vi "MPM_Sample.vi"() -> ()   [LabVIEW 2017]
uses:
  <vilib>/Utility/file.llb/Write To Spreadsheet File (DBL).vi
  <vilib>/Utility/file.llb/Write Delimited Spreadsheet (string).vi
  LV_IL_Sample/DLL/InstrumentDLL.dll
panel:
  out "MPM":refnum<k24>
  in  "选项卡控件":T1(tab)
  out "lblver4":string
  out "lblseri4":string
  out "lbltype4":string
  out "lblver3":string
  out "lblseri3":string
  out "lbltype3":string
  out "lblver2":string
  out "lblseri2":string
  out "lbltype2":string
  out "lblver1":string
  out "lblseri1":string
  out "lbltype1":string
  out "lblver0":string
  out "lblseri0":string
  out "lbltype0":string
  out "module count":string
  out "Product":string
  out "Serial":string
  out "F/ W Vesion":string
  in  "btnDisconnect":bool
  in  "btnConnect":bool
  in  "Portnumber":i32
  in  "Address/ComPort":string
  in  "Communication":T2(radio)
  in  "GetComport":bool
  in  "ComPort":u16(ring)
  in  "btnSplit":bool
  out "Address":dbl
  out "Board number":dbl
  in  "btnVisa":bool
  in  "Visa String":u16(ring)
  out "txtlan_port":string
  in  "btnGetPort":bool
  out "txtipaddress":string
  in  "btnGetIP":bool
  out "txtsyst_error":string
  in  "btnGetError":bool
  in  "btnGetWavelength":bool
  in  "txtwave_ch":i32 caption="Ch"
  in  "txtwave_slot":i32 caption="Slot"
  in  "btnZeroing":bool
  out "txtreadp_all":string caption="Read Power for each slot"
  in  "txtread_slotall":i32 caption="Slot"
  in  "btnSlot_Power":bool
  out "txt_readp_ch":dbl caption="Read Power for each ch"
  in  "txtread_ch":i32=1 caption="Ch"
  in  "txtread_slot":i32 caption="Slot"
  in  "btnSlot_Ch_Power":bool
  out "txtget_erange":dbl caption="Range for each ch"
  in  "txtget_rangech":i32=1 caption="Ch"
  in  "txtget_rangeslot":i32 caption="Slot"
  out "txtgetrmode":string caption="Range mode for \"READ\""
  in  "btnSlot_Ch_Range":bool
  in  "btnGet":bool
  out "txtget_unit":string caption="Unit"
  out "txtget_avg":dbl caption="Averaging time(msec)"
  out "txtget_wave":dbl caption="Wavelength(nm)"
  out "txtgetrang":i32 caption="Range All"
  in  "Ch":i32
  in  "Slot":i32
  in  "Range for each ch":i32
  in  "btnSetSlot":bool
  in  "Averaging time(msec)":dbl
  in  "btnSetAveraging":bool
  in  "btnSetUnit":bool
  in  "Unit":u16(ring) items=["dBm", "mW"]
  in  "btnSetRangeAll":bool
  in  "Range All":i32
  in  "btnSetRangeMode":bool
  in  "Range mode for \"READ\"":enum16{"Auto", "Manual"}(ring)
  in  "Wavelength(nm)":dbl
  in  "btnSetWavelength":bool
  in  "btnGetSlot":bool
  in  "txte_slot":i32 caption="Slot"
  in  "btnGetch":bool
  in  "txtlog_ch":i32 caption="Ch"
  in  "txtlog_slot":i32 caption="Slot"
  out "txtlog_status":string
  in  "btnStop":bool
  in  "btnStatus":bool
  in  "btnStart":bool
  in  "btnSetFreerun":bool
  in  "cmbfr_tin_mode":enum16{"Internal", "Extarnal"}(ring) caption="Trigger input mode"
  in  "txtfr_range":i32 caption="Range"
  in  "txtfr_point":i32 caption="number of point"
  in  "txtfr_ave":dbl caption="Averaging Time(msec)"
  in  "txtfr_wave":dbl caption="Wavelength(nm)"
  in  "btnSetSweep":bool
  in  "txtsm_range":i32 caption="Range"
  in  "cmbsm_rangemode":enum16{"Auto", "Manual"}(ring) caption="Range mode"
  in  "txtspeed":i32 caption="Speed(nm/sec)"
  in  "txtwavestep":dbl caption="Step wavelenght(nm)"
  in  "txtstopwave":dbl caption="Stop wavelenght(nm)"
  in  "txtstartwave":dbl caption="Start wavelength(nm)"
  in  "txtcon_range":i32 caption="Range"
  in  "cmbcon_rangemode":enum16{"Auto", "Manual"}(ring) caption="Range mode"
  in  "txtcon_point":i32 caption="number of point"
  in  "txtcon_ave":dbl caption="Averaging Time(msec)"
  in  "txtcon_wave":dbl caption="Wavelength(nm)"
  in  "btnSetConst":bool
  in  "btnGetParameter":bool
  out "txtg_speed":dbl caption="Sweep speed(nm)"
  out "txtg_stepwave":dbl caption="Step wavelength(nm)"
  out "txtg_stopwave":dbl caption="Stop wavelength(nm)"
  out "txtg_statwave":dbl caption="Start wavelength(nm)"
  out "txtg_wavelength":dbl caption="Wavelength(nm)"
  out "txtg_settingrange":string caption="Setting Range"
  out "txtg_tinmode":string caption="Trigger input mode"
  out "txtg_rangemode":string caption="Range mode"
  out "txtlog_mode":string caption="SweepMode"
  out "txtg_point":i32 caption="number of point"
  out "txtg_ave":dbl caption="Averaging time"
  # "0. Connect Tool"
  # "1. Connect"
  # "Communication setting"
  # "Information"
  # "Module Information"
  # "Slot0"
  # "Slot1"
  # "Slot2"
  # "Slot3"
  # "Slot4"
  # "Type"
  # "Serial"
  # "Version"
  # "Set"
  # "Get"
  # "Common function"
  # "Const Mode"
  # "Sweep Mode"
  # "FreerunMode"
  # "Common"
  # "Get Parameter"
  # "Sweep mode parameter"
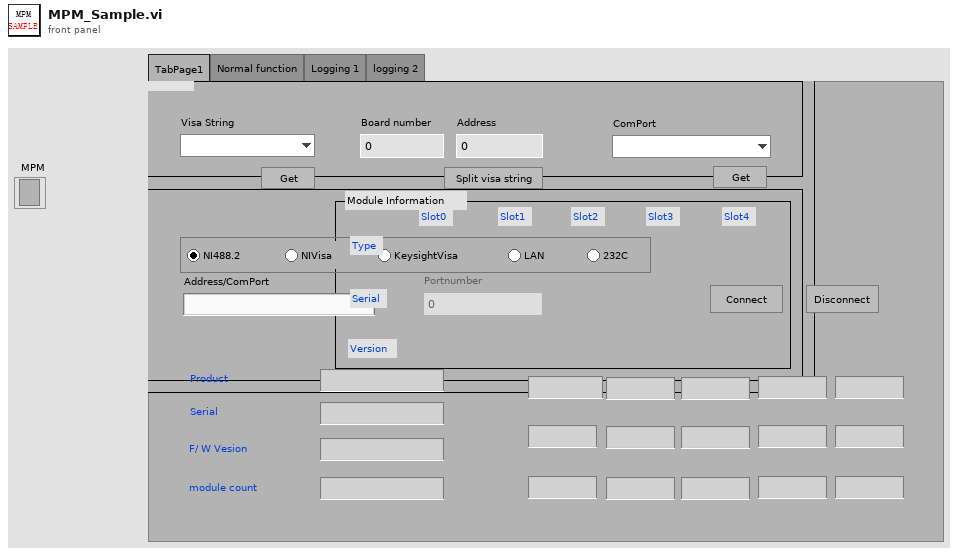
[diagram p1: front panel]
types:
  T1 = enum32{"TabPage1", "Normal function", "Logging 1", "logging 2"}
  T2 = enum32{"rdiNI488", "rdiNIvisa", "rdikeysightvisa", "rdiLAN", "rdi232C"}
  T3 = enum8{"Enabled", "Disabled", "Disabled and Grayed Out"}
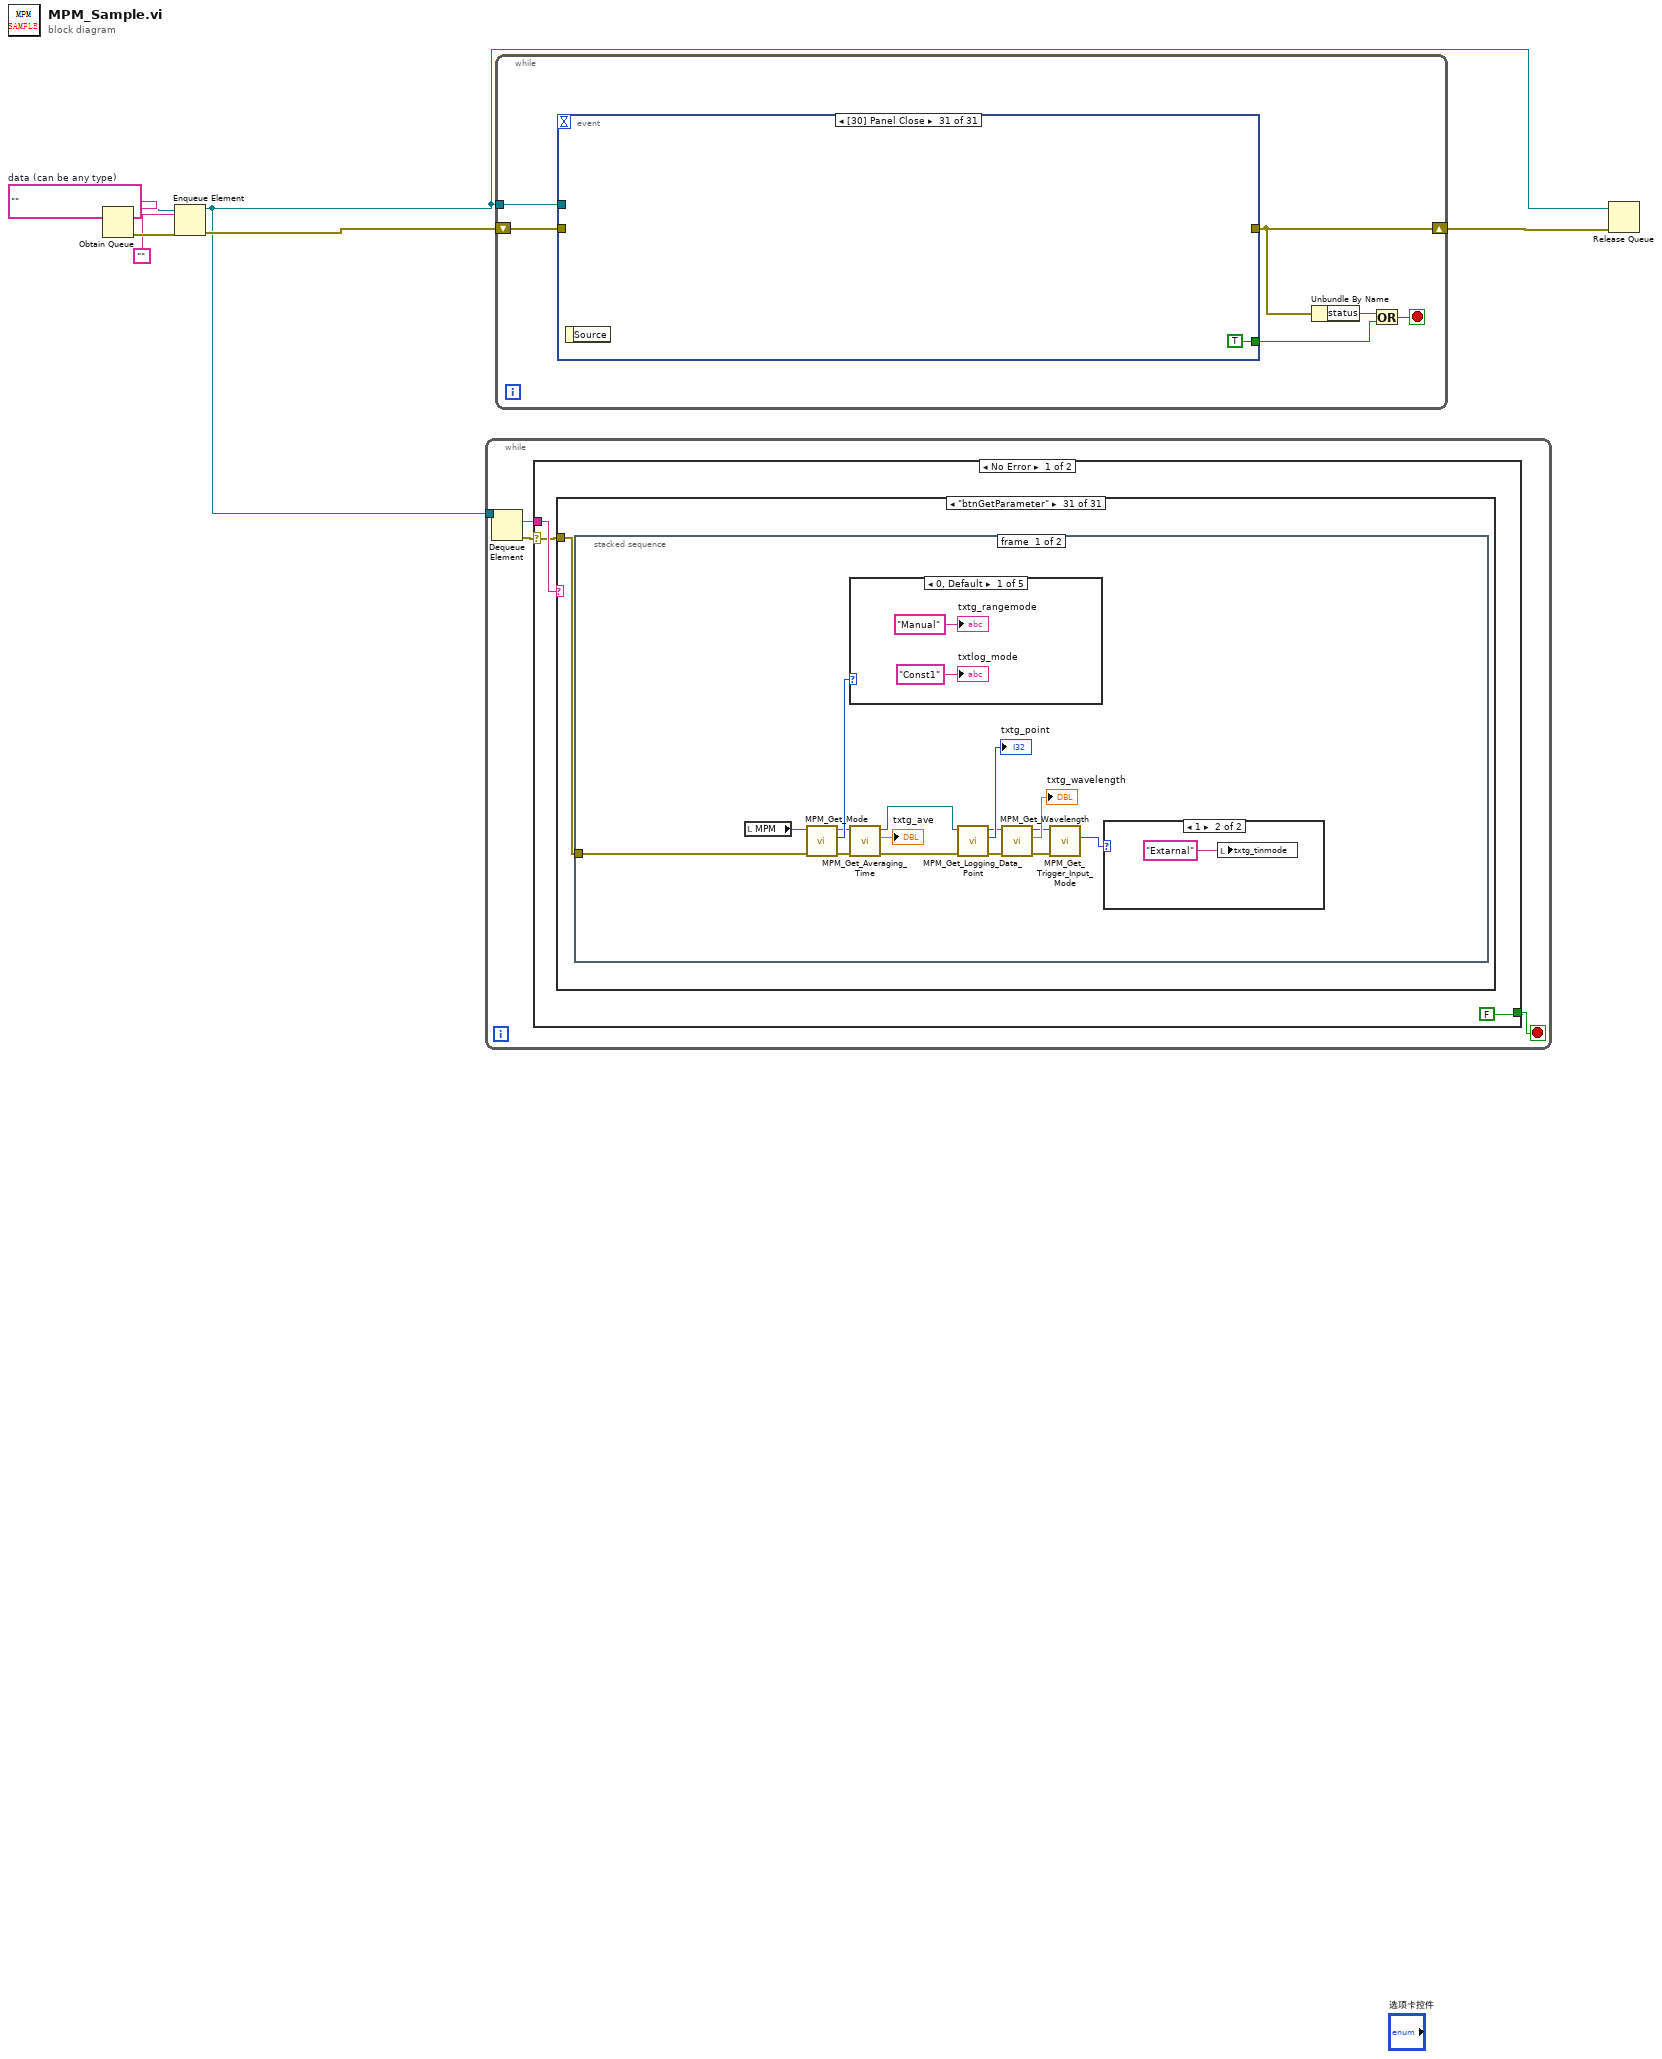
[diagram p0: block diagram]
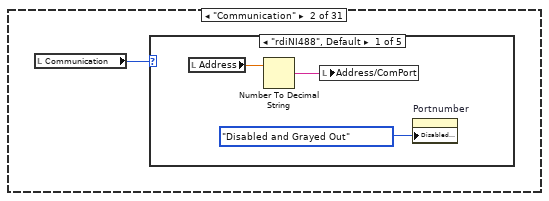
[diagram p3: hidden frame]
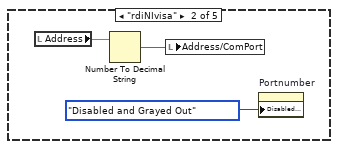
[diagram p4: hidden frame]
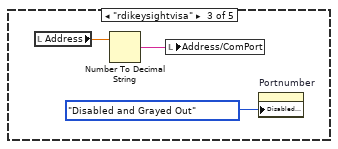
[diagram p5: hidden frame]
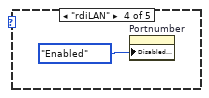
[diagram p6: hidden frame]
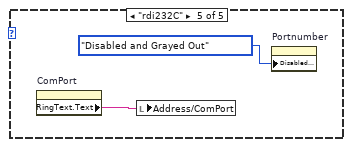
[diagram p7: hidden frame]
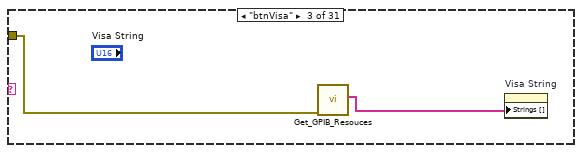
[diagram p8: hidden frame]
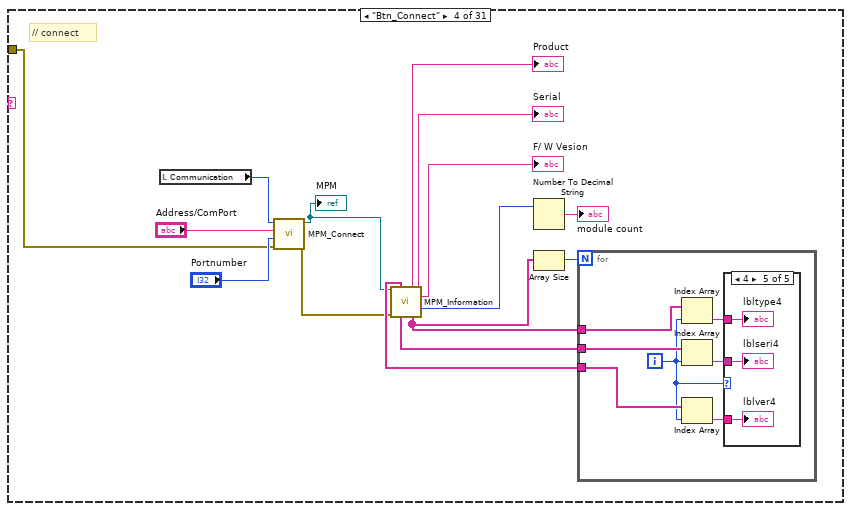
[diagram p9: hidden frame]
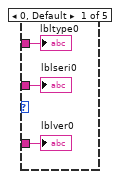
[diagram p10: hidden frame]
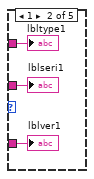
[diagram p11: hidden frame]
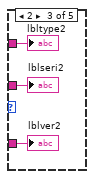
[diagram p12: hidden frame]
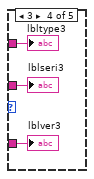
[diagram p13: hidden frame]
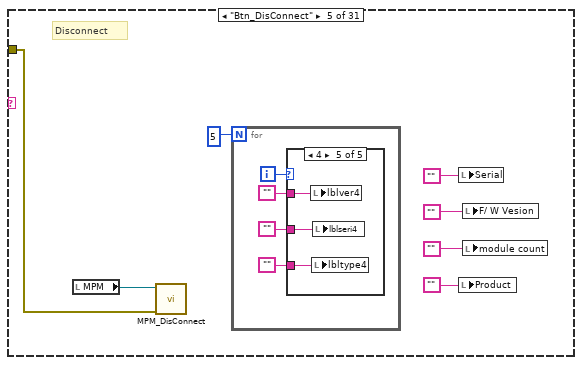
[diagram p14: hidden frame]
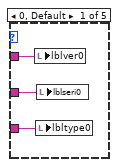
[diagram p15: hidden frame]
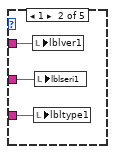
[diagram p16: hidden frame]
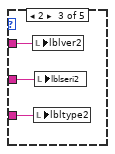
[diagram p17: hidden frame]
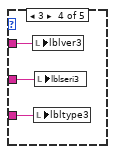
[diagram p18: hidden frame]
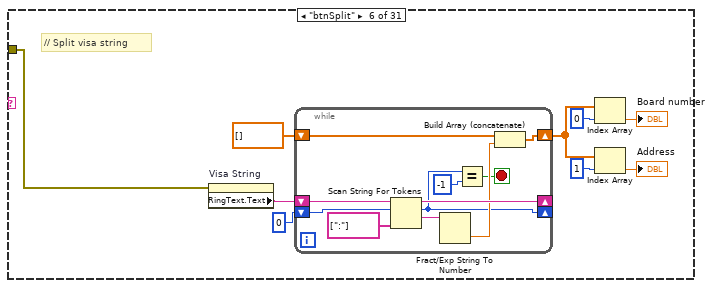
[diagram p19: hidden frame]
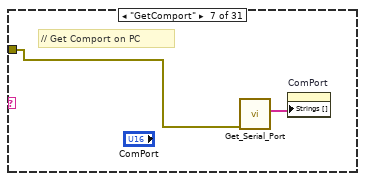
[diagram p20: hidden frame]
diagram:
  w4 = ""  # data (can be any type)
  n1 = Obtain Queue(element data type=w4) -> (queue out=w3:refnum<queue>, error out=w7:errorcluster)  [unwired: 4 in, 1 out]
  n2 = Enqueue Element(queue=w3, element="", error in (no error)=w7) -> (queue out=w1:refnum<queue>, error out=w6:errorcluster)  [unwired: 1 in, 1 out]
  n3 = while {
    tunnel: w1 -> [w11]
    stop <- w8 stop-if-true
    n4 = Dequeue Element(queue=w11) -> (element=w9:string, error out=w10:errorcluster)  [unwired: 2 in, 2 out]
    n5 = case shown="No Error" w10 {
      selector: w10 -> [w12 _]
      tunnel: w9 -> [w13 _]
      tunnel: [FALSE TRUE] -> w8
      frame No Error {
        n6 = case shown="\"btnGetParameter\"" w13 {
          tunnel: w12 -> [_ _ w28 w30 w67 w93 w113 w115 w133 w136 w139 w142 w147 w150 w169 w174 w179 w203 w205 w225 w228 w231 w238 w259 w283 w300 w302 w310 w313 w327 w340]
          frame "Load", Default {
          }
          frame "Communication" {
            n7 = local read "Communication"() -> (w15:T2)
            n8 = case shown="\"rdiNI488\", Default" w15 {
              frame "rdiNI488", Default {
                n9 = local read "Address"() -> (w16:dbl)
                n10 = Number To Decimal String(number=w16) -> (decimal integer string=w17:string)  [unwired: 1 in]
                n11 = local write "Address/ComPort"(w17) -> ()
                n12 = property on="Portnumber" class="DigNum (strict)"("DisabledEnum"=T3."Disabled and Grayed Out" ("禁用")) -> ()  [unwired: 2 in, 2 out]
              }
              frame "rdiNIvisa" {
                n13 = local read "Address"() -> (w19:dbl)
                n14 = Number To Decimal String(number=w19) -> (decimal integer string=w20:string)  [unwired: 1 in]
                n15 = local write "Address/ComPort"(w20) -> ()
                n16 = property on="Portnumber" class="DigNum (strict)"("DisabledEnum"=T3."Disabled and Grayed Out" ("禁用")) -> ()  [unwired: 2 in, 2 out]
              }
              frame "rdikeysightvisa" {
                n17 = local read "Address"() -> (w22:dbl)
                n18 = Number To Decimal String(number=w22) -> (decimal integer string=w23:string)  [unwired: 1 in]
                n19 = local write "Address/ComPort"(w23) -> ()
                n20 = property on="Portnumber" class="DigNum (strict)"("DisabledEnum"=T3."Disabled and Grayed Out" ("禁用")) -> ()  [unwired: 2 in, 2 out]
              }
              frame "rdiLAN" {
                n21 = property on="Portnumber" class="DigNum (strict)"("DisabledEnum"=T3."Enabled" ("禁用")) -> ()  [unwired: 2 in, 2 out]
              }
              frame "rdi232C" {
                n22 = property on="ComPort" class="Ring (strict)"() -> ("RingText.Text"=w26:string)  [unwired: 2 in, 2 out]
                n23 = local write "Address/ComPort"(w26) -> ()
                n24 = property on="Portnumber" class="DigNum (strict)"("DisabledEnum"=T3."Disabled and Grayed Out" ("禁用")) -> ()  [unwired: 2 in, 2 out]
              }
            }
          }
          frame "btnVisa" {
            n25 = call "Get_GPIB_Resouces.vi"("error in (no error)"=w28) -> ("Get_GPIB_Resources"=w29:string[])  [unwired: 8 in, 2 out]
            n26 = property on="Visa String" class="Ring (strict)"("Strings []"=w29) -> ()  [unwired: 2 in, 2 out]
          }
          frame "Btn_Connect" {
            # "// connect"
            n27 = local read "Communication"() -> (w32:T2)
            n28 = call "MPM_Connect.vi"("error in (no error)"=w30, "Portnumber"="Portnumber", "Address/ComPort"="Address/ComPort", "Communication"=w32) -> ("error out"=w33:errorcluster, "Reference out"=w31:refnum<k24>)  [unwired: 6 in]
            "MPM" <- w31
            n29 = call "MPM_Information.vi"(".NET Reference in"=w31, "error in (no error)"=w33) -> ("ModuleFW"=w37:string[], "ProductName"=→"Product":string, "FWversion"=→"F/ W Vesion":string, "SerialNumber"=→"Serial":string, "NumberofModule"=w43:i32, "ModuelSerial"=w38:string[], "ModuleType"=w35:string[])  [unwired: 5 in, 2 out]
            n30 = Number To Decimal String(number=w43) -> (decimal integer string=→"module count":string)  [unwired: 1 in]
            n31 = Array Size(array=w35) -> (size(s)=w34:i32)
            n32 = for {
              N: w34 -> [_]
              tunnel: w35 -> [w51]
              tunnel: w38 -> [w50]
              tunnel: w37 -> [w49]
              i -> [w48]
              n33 = Index Array(array=w51, index=w48) -> (element=w47:string)
              n34 = Index Array(array=w50, index=w48) -> (element=w46:string)
              n35 = Index Array(array=w49, index=w48) -> (element=w45:string)
              n36 = case shown="4" w48 {
                tunnel: w47 -> [w54 w57 w60 w63 w66]
                tunnel: w46 -> [w53 w56 w59 w62 w65]
                tunnel: w45 -> [w52 w55 w58 w61 w64]
                frame 0, Default {
                  "lbltype0" <- w54
                  "lblseri0" <- w53
                  "lblver0" <- w52
                }
                frame 1 {
                  "lbltype1" <- w57
                  "lblseri1" <- w56
                  "lblver1" <- w55
                }
                frame 2 {
                  "lbltype2" <- w60
                  "lblseri2" <- w59
                  "lblver2" <- w58
                }
                frame 3 {
                  "lbltype3" <- w63
                  "lblseri3" <- w62
                  "lblver3" <- w61
                }
                frame 4 {
                  "lbltype4" <- w66
                  "lblseri4" <- w65
                  "lblver4" <- w64
                }
              }
            }
          }
          frame "Btn_DisConnect" {
            # "Disconnect"
            n37 = local read "MPM"() -> (w73:refnum<k24>)
            n38 = call "MPM_DisConnect.vi"("error in (no error)"=w67, ".NET Reference in"=w73) -> ()  [unwired: 8 in, 2 out]
            n39 = for {
              N: 5 -> [_]
              i -> [w77]
              n40 = case shown="4" w77 {
                tunnel: "" -> [w80 w83 w86 w89 w92]
                tunnel: "" -> [w79 w82 w85 w88 w91]
                tunnel: "" -> [w78 w81 w84 w87 w90]
                frame 0, Default {
                  n41 = local write "lblver0"(w78) -> ()
                  n42 = local write "lbltype0"(w80) -> ()
                  n43 = local write "lblseri0"(w79) -> ()
                }
                frame 1 {
                  n44 = local write "lblver1"(w81) -> ()
                  n45 = local write "lbltype1"(w83) -> ()
                  n46 = local write "lblseri1"(w82) -> ()
                }
                frame 2 {
                  n47 = local write "lblver2"(w84) -> ()
                  n48 = local write "lbltype2"(w86) -> ()
                  n49 = local write "lblseri2"(w85) -> ()
                }
                frame 3 {
                  n50 = local write "lblver3"(w87) -> ()
                  n51 = local write "lbltype3"(w89) -> ()
                  n52 = local write "lblseri3"(w88) -> ()
                }
                frame 4 {
                  n53 = local write "lblver4"(w90) -> ()
                  n54 = local write "lbltype4"(w92) -> ()
                  n55 = local write "lblseri4"(w91) -> ()
                }
              }
            }
            n56 = local write "Serial"("") -> ()
            n57 = local write "Product"("") -> ()
            n58 = local write "F/ W Vesion"("") -> ()
            n59 = local write "module count"("") -> ()
          }
          frame "btnSplit" {
            # "// Split visa string"
            n60 = property on="Visa String" class="Ring (strict)"(error in=w93) -> ("RingText.Text"=w101:string)  [unwired: 1 in, 2 out]
            n61 = while {
              shift-right: [w110] -> _
              shift-left: w101 -> [w112]
              shift-right: [w105] -> _
              shift-left: 0 ("偏移量") -> [w111]
              shift-right: [w106] -> w97
              shift-left: dbl[] [] ("数组") -> [w107]
              stop <- w103 stop-if-true
              n62 = Scan String For Tokens(6:string[] [":"] ("分隔符(\\s,\\t,\\r,\\n)"), 8:w111, 9:w112) -> (1:w109:string, 2:w105:i32, 3:w110:string)  [unwired: 3 in, 1 out]
              n63 = Fract/Exp String To Number(string=w109) -> (number=w108:dbl)  [unwired: 3 in, 1 out]
              n64 = Equal?(x=w105, y=-1) -> (x = y?=w103:bool)
              n65 = Build Array (concatenate)(w107, w108) -> (w106:dbl[])
            }
            n66 = Index Array(array=w97, index=0 ("索引")) -> (element=→"Board number":dbl)
            n67 = Index Array(array=w97, index=1 ("索引")) -> (element=→"Address":dbl)
          }
          frame "GetComport" {
            # "// Get Comport on PC"
            n68 = call "Get_Serial_Port.vi"("error in (no error)"=w113) -> ("Get_Serial_Port"=w114:string[])  [unwired: 8 in, 2 out]
            n69 = property on="ComPort" class="Ring (strict)"("Strings []"=w114) -> ()  [unwired: 2 in, 2 out]
          }
          frame "btnSetRangeMode" {
            # "// Set Range Mode for \"READ\""
            n70 = property on="Range mode for \"READ\"" class="Enum (strict)"() -> ("RingText.Text"=w116:string)  [unwired: 2 in, 2 out]
            n71 = case shown="\"Manual\"" w116 {
              tunnel: w115 -> [w117 w125]
              frame "Manual" {
                n72 = stacked-sequence {
                  tunnel: w117 -> [_ w122]
                  frame #0 {
                    n73 = property on="Ch" class="DigNum (strict)"("DisabledEnum"=T3."Enabled" ("禁用")) -> ()  [unwired: 2 in, 2 out]
                    n74 = property on="Range for each ch" class="DigNum (strict)"("DisabledEnum"=T3."Enabled" ("禁用")) -> ()  [unwired: 2 in, 2 out]
                    n75 = property on="Slot" class="DigNum (strict)"("DisabledEnum"=T3."Enabled" ("禁用")) -> ()  [unwired: 2 in, 2 out]
                    n76 = property on="Range All" class="DigNum (strict)"("DisabledEnum"=T3."Enabled" ("禁用")) -> ()  [unwired: 2 in, 2 out]
                  }
                  frame #1 {
                    n77 = local read "Range mode for \"READ\""() -> (w124:enum16{"Auto", "Manual"})
                    n78 = local read "MPM"() -> (w123:refnum<k24>)
                    n79 = call "MPM_Set_Read_Rang_Mode.vi"("error in (no error)"=w122, "mode"=w124, ".NET Reference in"=w123) -> ()  [unwired: 7 in, 2 out]
                  }
                }
              }
              frame "Auto", Default {
                n80 = stacked-sequence {
                  tunnel: w125 -> [_ w130]
                  frame #0 {
                    n81 = property on="Slot" class="DigNum (strict)"("DisabledEnum"=T3."Disabled" ("禁用")) -> ()  [unwired: 2 in, 2 out]
                    n82 = property on="Range for each ch" class="DigNum (strict)"("DisabledEnum"=T3."Disabled" ("禁用")) -> ()  [unwired: 2 in, 2 out]
                    n83 = property on="Range All" class="DigNum (strict)"("DisabledEnum"=T3."Disabled" ("禁用")) -> ()  [unwired: 2 in, 2 out]
                    n84 = property on="Ch" class="DigNum (strict)"("DisabledEnum"=T3."Disabled" ("禁用")) -> ()  [unwired: 2 in, 2 out]
                  }
                  frame #1 {
                    n85 = local read "MPM"() -> (w132:refnum<k24>)
                    n86 = call "MPM_Set_Read_Rang_Mode.vi"("error in (no error)"=w130, "mode"="Range mode for \"READ\"", ".NET Reference in"=w132) -> ()  [unwired: 7 in, 2 out]
                  }
                }
              }
            }
          }
          frame "btnSetRangeAll" {
            # "// Set range for munal range\n            // MPM-211/212 : 1～5 MPM213 : 1～4　　MPM215 : Nothing"
            n87 = local read "MPM"() -> (w135:refnum<k24>)
            n88 = call "MPM_Set_Range.vi"("error in (no error)"=w133, "Range All"="Range All", ".NET Reference in"=w135) -> ()  [unwired: 7 in, 2 out]
          }
          frame "btnSetWavelength" {
            # "// Set Wavelength(nm)"
            n89 = local read "MPM"() -> (w138:refnum<k24>)
            n90 = call "MPM_Set_Wavelength.vi"("error in (no error)"=w136, "Wavelength(nm)"="Wavelength(nm)", ".NET Reference in"=w138) -> ()  [unwired: 7 in, 2 out]
          }
          frame "btnSetUnit" {
            # "// Set Power unit"
            n91 = local read "MPM"() -> (w141:refnum<k24>)
            n92 = call "MPM_Set_Unit.vi"("error in (no error)"=w139, "unit"="Unit", ".NET Reference in"=w141) -> ()  [unwired: 7 in, 2 out]
          }
          frame "btnSetAveraging" {
            # "// Set Averaging Time(mse)\n            // MPM can set 0.01msec～10000msec"
            n93 = local read "MPM"() -> (w144:refnum<k24>)
            n94 = call "MPM_Set_Averaging_Time.vi"("error in (no error)"=w142, "Averaging time(msec)"="Averaging time(msec)", ".NET Reference in"=w144) -> ()  [unwired: 7 in, 2 out]
          }
          frame "btnSetSlot" {
            # "// Set Range for each ch"
            n95 = local read "MPM"() -> (w149:refnum<k24>)
            n96 = call "MPM_Set_Range_Each_Channel.vi"("Range for each ch"="Range for each ch", "error in (no error)"=w147, "Ch"="Ch", "Slot"="Slot", ".NET Reference in"=w149) -> ()  [unwired: 5 in, 2 out]
          }
          frame "btnGet" {
            # "// Get normal function parameter"
            n97 = local read "MPM"() -> (w164:refnum<k24>)
            n98 = call "MPM_Get_Read_Range_Mode.vi"("error in (no error)"=w150, ".NET Reference in"=w164) -> ("error out"=w162:errorcluster, "mode"=w151:enum16{"Manual", "Auto"}, "Reference out"=w163:refnum<k24>)  [unwired: 7 in]
            n99 = case shown="\"Auto\"" w151 {
              frame "Manual", Default {
                n100 = local write "txtgetrmode"("Manual") -> ()
              }
              frame "Auto" {
                "txtgetrmode" <- "Auto"
              }
            }
            n101 = call "MPM_Get_Range.vi"("error in (no error)"=w162, ".NET Reference in"=w163) -> ("error out"=w160:errorcluster, "range out"=→"txtgetrang":i32, "Reference out"=w161:refnum<k24>)  [unwired: 7 in]
            n102 = call "MPM_Get_Wavelength.vi"("error in (no error)"=w160, ".NET Reference in"=w161) -> ("error out"=w157:errorcluster, "wave out"=→"txtget_wave":dbl, "Reference out"=w158:refnum<k24>)  [unwired: 7 in]
            n103 = call "MPM_Get_Averaging_Time.vi"("error in (no error)"=w157, ".NET Reference in"=w158) -> ("error out"=w154:errorcluster, "time out"=→"txtget_avg":dbl, "Reference out"=w155:refnum<k24>)  [unwired: 7 in]
            n104 = call "MPM_Get_Unit.vi"("error in (no error)"=w154, ".NET Reference in"=w155) -> ("unit"=w152:enum16{"dBmA, dBm", "mW, mA"})  [unwired: 7 in, 2 out]
            n105 = case shown="\"mW, mA\"" w152 {
              frame "dBmA, dBm", Default {
                n106 = local write "txtget_unit"("dBm") -> ()
              }
              frame "mW, mA" {
                "txtget_unit" <- "mW"
              }
            }
          }
          frame "btnSlot_Ch_Range" {
            # "// Get Range for each ch"
            n107 = local read "MPM"() -> (w173:refnum<k24>)
            n108 = call "MPM_Get_Range_Each_for_Channel.vi"("error in (no error)"=w169, "channelNumber"="txtget_rangech", "moduleNumber"="txtget_rangeslot", ".NET Reference in"=w173) -> ("range out"=→"txtget_erange":i32)  [unwired: 5 in, 2 out]
          }
          frame "btnSlot_Ch_Power" {
            # "// Read Power for each ch"
            n109 = local read "MPM"() -> (w178:refnum<k24>)
            n110 = call "MPM_Get_READ_Power_for_Channel.vi"("error in (no error)"=w174, "channelNumber"="txtread_ch", "moduleNumber"="txtread_slot", ".NET Reference in"=w178) -> ("power out"=→"txt_readp_ch":dbl)  [unwired: 5 in, 2 out]
          }
          frame "btnSlot_Power" {
            # "// Read Power for Slot"
            n111 = local read "MPM"() -> (w202:refnum<k24>)
            n112 = call "MPM_Get_READ_Power_for_Module.vi"("error in (no error)"=w179, "moduleNumber"="txtread_slotall", ".NET Reference in"=w202) -> ("powers out"=w184:dbl[])  [unwired: 6 in, 2 out]
            n113 = Index Array(array=w184, index #1=0 ("索引"), index #2=1 ("索引"), index #3=2 ("索引"), index #4=3 ("索引")) -> (element #1=w193:dbl, element #2=w194:dbl, element #3=w195:dbl, element #4=w196:dbl)
            n114 = Number To Fractional String(number=w193, precision (6)=i16 3 ("精度(6)")) -> (F-format string=w191:string)  [unwired: 2 in]
            n115 = Number To Fractional String(number=w194, precision (6)=i16 3 ("精度(6)")) -> (F-format string=w189:string)  [unwired: 2 in]
            n116 = Number To Fractional String(number=w195, precision (6)=i16 3 ("精度(6)")) -> (F-format string=w187:string)  [unwired: 2 in]
            n117 = Number To Fractional String(number=w196, precision (6)=i16 3 ("精度(6)")) -> (F-format string=w185:string)  [unwired: 2 in]
            n118 = Concatenate Strings(w191, "," ("字符串"), w189, "," ("字符串"), w187, "," ("字符串"), w185) -> (→"txtreadp_all":string)
          }
          frame "btnZeroing" {
            # "// Zeroing function"
            n119 = local read "MPM"() -> (w204:refnum<k24>)
            n120 = call "MPM_Zeroing.vi"("error in (no error)"=w203, ".NET Reference in"=w204) -> ()  [unwired: 8 in, 2 out]
          }
          frame "btnGetWavelength" {
            # "// Get Wavelength Sencitvity data for each ch"
            n121 = local read "MPM"() -> (w214:refnum<k24>)
            n122 = call "MPM_Get_Wavelength_Senctivity_Data.vi"("error in (no error)"=w205, "channelNumber"="txtwave_ch", "moduleNumber"="txtwave_slot", ".NET Reference in"=w214) -> ("offsetpower out"=w208:sgl[], "wavedata out"=w207:dbl[])  [unwired: 4 in, 2 out]
            n123 = Array Size(array=w207) -> (size(s)=w212:i32)
            n124 = for {
              N: w212 -> [_]
              tunnel: w208 -> [w224]
              tunnel: w207 -> [w223]
              tunnel: [w215] -> w211
              i -> [w222]
              n125 = Index Array(array=w223, index=w222) -> (element=w221:dbl)
              n126 = Index Array(array=w224, index=w222) -> (element=w220:sgl)
              n127 = Number To Hexadecimal String(2:w221) -> (0:w219:string)  [unwired: 1 in]
              n128 = Number To Hexadecimal String(2:w220) -> (0:w218:string)  [unwired: 1 in]
              n129 = Concatenate Strings(w219, "，" ("字符串"), w218) -> (w216:string)
              n130 = Initialize Array(w216) -> (w215:string[])  [unwired: 1 in]
            }
            n131 = call-poly <vilib>:"Write Delimited Spreadsheet.vi"("format (%s)"="%s", "1D data"=w211, "transpose? (no:F)"=FALSE ("transpose? (F)")) -> ()  [unwired: 11 in, 2 out]
          }
          frame "btnGetError" {
            # "// Get MPM error code"
            n132 = local read "MPM"() -> (w227:refnum<k24>)
            n133 = call "MPM_Get_System_Error.vi"("error in (no error)"=w225, ".NET Reference in"=w227) -> ("error"=→"txtsyst_error":string)  [unwired: 7 in, 2 out]
          }
          frame "btnGetIP" {
            n134 = local read "MPM"() -> (w230:refnum<k24>)
            n135 = call "MPM_Get_IPAddress.vi"("error in (no error)"=w228, ".NET Reference in"=w230) -> ("address out"=→"txtipaddress":string)  [unwired: 7 in, 2 out]
          }
          frame "btnGetPort" {
            n136 = local read "MPM"() -> (w234:refnum<k24>)
            n137 = call "MPM_Get_LAN_PortNumber.vi"("error in (no error)"=w231, ".NET Reference in"=w234) -> ("port out"=w232:i32)  [unwired: 7 in, 2 out]
            n138 = Number To Decimal String(number=w232) -> (decimal integer string=→"txtlan_port":string)  [unwired: 1 in]
          }
          frame "btnSetConst" {
            w243 = 1 items=["Internal", "Extarnal"] ("mode")
            n139 = local read "MPM"() -> (w236:refnum<k24>)
            n140 = call "MPM_Set_Averaging_Time.vi"("error in (no error)"=w238, "Averaging time(msec)"="txtcon_ave", ".NET Reference in"=w236) -> ("error out"=w241:errorcluster, "Reference out"=w246:refnum<k24>)  [unwired: 7 in]
            n141 = call "MPM_Set_Logging_Data_Point.vi"("error in (no error)"=w241, "count"="txtcon_point", ".NET Reference in"=w246) -> ("error out"=w240:errorcluster, "Reference out"=w245:refnum<k24>)  [unwired: 7 in]
            n142 = call "MPM_Set_Wavelength.vi"("error in (no error)"=w240, "Wavelength(nm)"="txtcon_wave", ".NET Reference in"=w245) -> ("error out"=w239:errorcluster, "Reference out"=w242:refnum<k24>)  [unwired: 7 in]
            n143 = call "MPM_Set_Trigger_Input_Mode.vi"("error in (no error)"=w239, "mode"=w243, ".NET Reference in"=w242) -> ("error out"=w237:errorcluster, "Reference out"=w235:refnum<k24>)  [unwired: 7 in]
            n144 = case shown="\"Auto\", Default" "cmbcon_rangemode" {
              tunnel: w235 -> [w251 w258]
              tunnel: w237 -> [w250 w253]
              frame "Auto", Default {
                w252 = 2 items=["ManualRangeConstant", "ManualRangeSweep", "AutoRangeConstant", "AutoRangeSweep", "Freerun"] ("mode")
                n145 = call "MPM_Set_Mode.vi"("error in (no error)"=w250, "mode"=w252, ".NET Reference in"=w251) -> ()  [unwired: 7 in, 2 out]
              }
              frame "Manual" {
                w257 = 0 items=["ManualRangeConstant", "ManualRangeSweep", "AutoRangeConstant", "AutoRangeSweep", "Freerun"] ("mode")
                n146 = call "MPM_Set_Mode.vi"("error in (no error)"=w253, "mode"=w257, ".NET Reference in"=w258) -> ("error out"=w254:errorcluster, "Reference out"=w255:refnum<k24>)  [unwired: 7 in]
                n147 = call "MPM_Set_Range.vi"("error in (no error)"=w254, "Range All"="txtcon_range", ".NET Reference in"=w255) -> ()  [unwired: 7 in, 2 out]
              }
            }
          }
          frame "btnSetSweep" {
            w263 = 1 items=["Internal", "Extarnal"] ("mode")
            n148 = local read "MPM"() -> (w262:refnum<k24>)
            n149 = call "MPM_Set_Trigger_Input_Mode.vi"("error in (no error)"=w259, "mode"=w263, ".NET Reference in"=w262) -> ("error out"=w264:errorcluster, "Reference out"=w265:refnum<k24>)  [unwired: 7 in]
            n150 = call "MPM_Set_Sweep_Wavelength.vi"("wavestep"="txtwavestep", "error in (no error)"=w264, "stopwave"="txtstopwave", "startwave"="txtstartwave", ".NET Reference in"=w265) -> ("error out"=w268:errorcluster, "Reference out"=w269:refnum<k24>)  [unwired: 5 in]
            n151 = call "MPM_Set_Sweep_Speed.vi"("error in (no error)"=w268, "speed"="txtspeed", ".NET Reference in"=w269) -> ("error out"=w260:errorcluster, "Reference out"=w261:refnum<k24>)  [unwired: 7 in]
            n152 = case shown="\"Auto\", Default" "cmbsm_rangemode" {
              tunnel: w261 -> [w274 w280]
              tunnel: w260 -> [w273 w276]
              frame "Auto", Default {
                w275 = 3 items=["ManualRangeConstant", "ManualRangeSweep", "AutoRangeConstant", "AutoRangeSweep", "Freerun"] ("mode")
                n153 = call "MPM_Set_Mode.vi"("error in (no error)"=w273, "mode"=w275, ".NET Reference in"=w274) -> ()  [unwired: 7 in, 2 out]
              }
              frame "Manual" {
                w281 = 1 items=["ManualRangeConstant", "ManualRangeSweep", "AutoRangeConstant", "AutoRangeSweep", "Freerun"] ("mode")
                n154 = call "MPM_Set_Mode.vi"("error in (no error)"=w276, "mode"=w281, ".NET Reference in"=w280) -> ("error out"=w277:errorcluster, "Reference out"=w278:refnum<k24>)  [unwired: 7 in]
                n155 = call "MPM_Set_Range.vi"("error in (no error)"=w277, "Range All"="txtsm_range", ".NET Reference in"=w278) -> ()  [unwired: 7 in, 2 out]
              }
            }
          }
          frame "btnSetFreerun" {
            w298 = 4 items=["ManualRangeConstant", "ManualRangeSweep", "AutoRangeConstant", "AutoRangeSweep", "Freerun"] ("mode")
            n156 = local read "MPM"() -> (w299:refnum<k24>)
            n157 = call "MPM_Set_Mode.vi"("error in (no error)"=w283, "mode"=w298, ".NET Reference in"=w299) -> ("error out"=w287:errorcluster, "Reference out"=w297:refnum<k24>)  [unwired: 7 in]
            n158 = call "MPM_Set_Range.vi"("error in (no error)"=w287, "Range All"="txtfr_range", ".NET Reference in"=w297) -> ("error out"=w286:errorcluster, "Reference out"=w295:refnum<k24>)  [unwired: 7 in]
            n159 = call "MPM_Set_Averaging_Time.vi"("error in (no error)"=w286, "Averaging time(msec)"="txtfr_ave", ".NET Reference in"=w295) -> ("error out"=w288:errorcluster, "Reference out"=w293:refnum<k24>)  [unwired: 7 in]
            n160 = call "MPM_Set_Logging_Data_Point.vi"("error in (no error)"=w288, "count"="txtfr_point", ".NET Reference in"=w293) -> ("error out"=w285:errorcluster, "Reference out"=w290:refnum<k24>)  [unwired: 7 in]
            n161 = call "MPM_Set_Wavelength.vi"("error in (no error)"=w285, "Wavelength(nm)"="txtfr_wave", ".NET Reference in"=w290) -> ("error out"=w284:errorcluster, "Reference out"=w289:refnum<k24>)  [unwired: 7 in]
            n162 = call "MPM_Set_Trigger_Input_Mode.vi"("error in (no error)"=w284, "mode"="cmbfr_tin_mode", ".NET Reference in"=w289) -> ()  [unwired: 7 in, 2 out]
          }
          frame "btnStart" {
            n163 = local read "MPM"() -> (w301:refnum<k24>)
            n164 = call "MPM_Logging_Start.vi"("error in (no error)"=w300, ".NET Reference in"=w301) -> ()  [unwired: 8 in, 2 out]
          }
          frame "btnStatus" {
            n165 = local read "MPM"() -> (w309:refnum<k24>)
            n166 = call "MPM_Get_Logging_Status.vi"("error in (no error)"=w302, ".NET Reference in"=w309) -> ("count out"=w304:i32, "status out"=w303:i32)  [unwired: 6 in, 2 out]
            n167 = Number To Decimal String(number=w303) -> (decimal integer string=w307:string)  [unwired: 1 in]
            n168 = Number To Decimal String(number=w304) -> (decimal integer string=w306:string)  [unwired: 1 in]
            n169 = Concatenate Strings(w307, "," ("字符串"), w306) -> (→"txtlog_status":string)
          }
          frame "btnStop" {
            n170 = local read "MPM"() -> (w311:refnum<k24>)
            n171 = call "MPM_Logging_Stop.vi"("error in (no error)"=w310, ".NET Reference in"=w311) -> ()  [unwired: 8 in, 2 out]
          }
          frame "btnGetch" {
            n172 = local read "MPM"() -> (w317:refnum<k24>)
            n173 = call "MPM_Get_Each_Channel_Logdata.vi"("error in (no error)"=w313, "channelNumber"="txtlog_ch", "moduleNumber"="txtlog_slot", ".NET Reference in"=w317) -> ("data out"=w312:sgl[])  [unwired: 5 in, 2 out]
            n174 = call-poly <vilib>:"Write To Spreadsheet File.vi"("transpose? (no:F)"=TRUE, "1D data"=w312) -> ()  [unwired: 6 in, 1 out]
          }
          frame "btnGetSlot" {
            n175 = local read "MPM"() -> (w332:refnum<k24>)
            n176 = call "MPM_Get_Each_Module_Loggdata.vi"("error in (no error)"=w327, "moduleNumber"="txte_slot", ".NET Reference in"=w332) -> ("data out"=w325:sgl[][])  [unwired: 6 in, 2 out]
            n177 = Array Size(array=w325) -> (size(s)=w329:i32[])
            n178 = Index Array(array=w329, index=0 ("索引")) -> (element=w323:i32)
            n179 = Number To Fractional String ("数値を小数文字列に変換")(number=w325, precision (6)=i16 6 ("精度(6)")) -> (F-format string=w322:string[][])  [unwired: 2 in]
            n180 = for {
              N: w323 -> [_]
              shift-right: [w333] -> w326
              shift-left: string[] [] -> [w335]
              i -> [w339]
              n181 = Increment(x=w339) -> (x+1=w338:i32)
              n182 = Format Into String(format string="%d", initial string="Ch", w338) -> (resulting string=w334:string)  [unwired: 1 in, 1 out]
              n183 = Build Array (concatenate)(w335, w334) -> (w333:string[])
            }
            n184 = Transpose 2D Array(2D array=w322) -> (transposed array=w321:string[][])
            n185 = Build Array (concatenate)(w326, w321) -> (w320:string[][])
            n186 = call-poly <vilib>:"Write Delimited Spreadsheet.vi"("format (%s)"="%s", "2D data"=w320, "delimiter (\\t)"="," ("delimiter (\\t)")) -> ()  [unwired: 11 in, 2 out]
          }
          frame "btnGetParameter" {
            n187 = stacked-sequence {
              tunnel: w340 -> [w341 w368]
              frame #0 {
                n188 = local read "MPM"() -> (w355:refnum<k24>)
                n189 = call "MPM_Get_Mode.vi"("error in (no error)"=w341, ".NET Reference in"=w355) -> ("error out"=w352:errorcluster, "mode"=w354:i32, "Reference out"=w353:refnum<k24>)  [unwired: 7 in]
                n190 = case shown="0, Default" w354 {
                  frame 0, Default {
                    "txtg_rangemode" <- "Manual"
                    "txtlog_mode" <- "Const1"
                  }
                  frame 1 {
                    n191 = local write "txtlog_mode"("Sweep1") -> ()
                    n192 = local write "txtg_rangemode"("Manual") -> ()
                  }
                  frame 2 {
                    n193 = local write "txtg_rangemode"("Auto") -> ()
                    n194 = local write "txtlog_mode"("Const2") -> ()
                  }
                  frame 3 {
                    n195 = local write "txtg_rangemode"("Auto") -> ()
                    n196 = local write "txtlog_mode"("Sweep2") -> ()
                  }
                  frame 4 {
                    n197 = local write "txtlog_mode"("Freerun") -> ()
                    n198 = local write "txtg_rangemode"("Manual") -> ()
                  }
                }
                n199 = call "MPM_Get_Averaging_Time.vi"("error in (no error)"=w352, ".NET Reference in"=w353) -> ("error out"=w344:errorcluster, "time out"=→"txtg_ave":dbl, "Reference out"=w345:refnum<k24>)  [unwired: 7 in]
                n200 = call "MPM_Get_Logging_Data_Point.vi"("error in (no error)"=w344, ".NET Reference in"=w345) -> ("error out"=w342:errorcluster, "count out"=→"txtg_point":i32, "Reference out"=w343:refnum<k24>)  [unwired: 7 in]
                n201 = call "MPM_Get_Wavelength.vi"("error in (no error)"=w342, ".NET Reference in"=w343) -> ("error out"=w347:errorcluster, "wave out"=→"txtg_wavelength":dbl, "Reference out"=w348:refnum<k24>)  [unwired: 7 in]
                n202 = call "MPM_Get_Trigger_Input_Mode.vi"("error in (no error)"=w347, ".NET Reference in"=w348) -> ("mode"=w349:i32)  [unwired: 7 in, 2 out]
                n203 = case shown="1" w349 {
                  frame 0, Default {
                    "txtg_tinmode" <- "Internal"
                  }
                  frame 1 {
                    n204 = local write "txtg_tinmode"("Extarnal") -> ()
                  }
                }
              }
              frame #1 {
                n205 = local read "txtg_rangemode"() -> (w371:string)
                n206 = local read "txtlog_mode"() -> (w372:string)
                n207 = Equal?(x=w371, y="Manual") -> (x = y?=w369:bool)
                n208 = Match Pattern(string=w372, regular expression="Sweep") -> (offset past match=w374:i32)  [unwired: 1 in, 3 out]
                n209 = case shown="True" w369 {
                  tunnel: w368 -> [_ w378]
                  frame False {
                    "txtg_settingrange" <- ""
                  }
                  frame True {
                    n210 = local read "MPM"() -> (w380:refnum<k24>)
                    n211 = call "MPM_Get_Range.vi"("error in (no error)"=w378, ".NET Reference in"=w380) -> ("range out"=w379:i32)  [unwired: 7 in, 2 out]
                    n212 = Number To Decimal String(number=w379) -> (decimal integer string=w381:string)  [unwired: 1 in]
                    n213 = local write "txtg_settingrange"(w381) -> ()
                  }
                }
                n214 = Not Equal?(x=w374, y=-1) -> (x != y?=w376:bool)
                n215 = case shown="False" w376 {
                  tunnel: w368 -> [w382 _]
                  frame False {
                    n216 = local read "MPM"() -> (w389:refnum<k24>)
                    n217 = call "MPM_Get_Sweep_Wavelength.vi"("error in (no error)"=w382, ".NET Reference in"=w389) -> ("error out"=w384:errorcluster, "stopwave out"=→"txtg_stopwave":dbl, "startwave out"=→"txtg_statwave":dbl, "Reference out"=w385:refnum<k24>, "stepwave out"=→"txtg_stepwave":dbl)  [unwired: 5 in]
                    n218 = call "MPM_Get_Sweep_Speed.vi"("error in (no error)"=w384, ".NET Reference in"=w385) -> ("speed"=→"txtg_speed":dbl)  [unwired: 7 in, 2 out]
                  }
                  frame True {
                    n219 = Decimal String To Number(string="") -> (number=w391:i32)  [unwired: 2 in, 1 out]
                    n220 = local write "txtg_ave"(w391) -> ()
                  }
                }
              }
            }
          }
        }
      }
      frame Error {
      }
    }
  }
  n221 = while {
    tunnel: w1 -> [w393]
    shift-right: [w395] -> w5
    shift-left: w6 -> [w394]
    stop <- w396 stop-if-true
    n222 = event shown="[30] Panel Close" {
      selector: _ -> [_ _ _ _ _ _ _ _ _ _ _ _ _ _ _ _ _ _ _ _ _ _ _ _ _ _ _ _ _ _ _]
      dyn-events: _ -> [_ _ _ _ _ _ _ _ _ _ _ _ _ _ _ _ _ _ _ _ _ _ _ _ _ _ _ _ _ _ _]
      timeout: _ -> [_ _ _ _ _ _ _ _ _ _ _ _ _ _ _ _ _ _ _ _ _ _ _ _ _ _ _ _ _ _ _]
      tunnel: w394 -> [w402 w404 w409 w414 w418 w420 w425 w428 w432 w436 w440 w444 w448 w452 w456 w460 w464 w468 w472 w476 w480 w484 w488 w492 w496 w500 w504 w508 w512 w516 _]
      tunnel: [w401 w406 w408 w412 w416 w422 w424 w430 w434 w438 w442 w446 w450 w454 w458 w462 w466 w470 w474 w478 w482 w486 w490 w494 w498 w502 w506 w510 w514 w518 _] -> w395
      tunnel: [FALSE ("stop") _ _ _ _ _ _ _ _ _ _ _ _ _ _ _ _ _ _ _ _ _ _ _ _ _ _ _ _ _ TRUE ("stop")] -> w397
      tunnel: w393 -> [w403 w405 w410 w413 w417 w421 w426 w429 w433 w437 w441 w445 w449 w453 w457 w461 w465 w469 w473 w477 w481 w485 w489 w493 w497 w501 w505 w509 w513 w517 _]
      event "btnConnect": Value Change {
        n223 = event-data() -> ()  [unwired: 1 in, 1 out]
        n224 = Enqueue Element(queue=w403, element="Btn_Connect" ("元素"), error in (no error)=w402) -> (error out=w401:errorcluster)  [unwired: 1 in, 2 out]
      }
      event "btnDisconnect": Value Change {
        n225 = event-data() -> ()  [unwired: 1 in, 1 out]
        n226 = Enqueue Element(queue=w405, element="Btn_DisConnect" ("元素"), error in (no error)=w404) -> (error out=w406:errorcluster)  [unwired: 1 in, 2 out]
      }
      event "btnSplit": Value Change {
        n227 = event-data() -> ()  [unwired: 1 in, 1 out]
        n228 = Enqueue Element(queue=w410, element="btnSplit" ("元素"), error in (no error)=w409) -> (error out=w408:errorcluster)  [unwired: 1 in, 2 out]
      }
      event "GetComport": Value Change {
        n229 = event-data() -> ()  [unwired: 1 in, 1 out]
        n230 = Enqueue Element(queue=w413, element="GetComport" ("元素"), error in (no error)=w414) -> (error out=w412:errorcluster)  [unwired: 1 in, 2 out]
      }
      event "btnSetRangeMode": Value Change {
        n231 = event-data() -> ()  [unwired: 1 in, 1 out]
        n232 = Enqueue Element(queue=w417, element="btnSetRangeMode" ("元素"), error in (no error)=w418) -> (error out=w416:errorcluster)  [unwired: 1 in, 2 out]
      }
      event "btnSetRangeAll": Value Change {
        n233 = event-data() -> ()  [unwired: 1 in, 1 out]
        n234 = Enqueue Element(queue=w421, element="btnSetRangeAll" ("元素"), error in (no error)=w420) -> (error out=w422:errorcluster)  [unwired: 1 in, 2 out]
      }
      event "btnSetWavelength": Value Change {
        n235 = event-data() -> ()  [unwired: 1 in, 1 out]
        n236 = Enqueue Element(queue=w426, element="btnSetWavelength" ("元素"), error in (no error)=w425) -> (error out=w424:errorcluster)  [unwired: 1 in, 2 out]
      }
      event "btnSetUnit": Value Change {
        n237 = event-data() -> ()  [unwired: 1 in, 1 out]
        n238 = Enqueue Element(queue=w429, element="btnSetUnit" ("元素"), error in (no error)=w428) -> (error out=w430:errorcluster)  [unwired: 1 in, 2 out]
      }
      event "btnSetAveraging": Value Change {
        n239 = event-data() -> ()  [unwired: 1 in, 1 out]
        n240 = Enqueue Element(queue=w433, element="btnSetAveraging" ("元素"), error in (no error)=w432) -> (error out=w434:errorcluster)  [unwired: 1 in, 2 out]
      }
      event "btnSetSlot": Value Change {
        n241 = event-data() -> ()  [unwired: 1 in, 1 out]
        n242 = Enqueue Element(queue=w437, element="btnSetSlot" ("元素"), error in (no error)=w436) -> (error out=w438:errorcluster)  [unwired: 1 in, 2 out]
      }
      event "btnGet": Value Change {
        n243 = event-data() -> ()  [unwired: 1 in, 1 out]
        n244 = Enqueue Element(queue=w441, element="btnGet" ("元素"), error in (no error)=w440) -> (error out=w442:errorcluster)  [unwired: 1 in, 2 out]
      }
      event "btnSlot_Ch_Range": Value Change {
        n245 = event-data() -> ()  [unwired: 1 in, 1 out]
        n246 = Enqueue Element(queue=w445, element="btnSlot_Ch_Range" ("元素"), error in (no error)=w444) -> (error out=w446:errorcluster)  [unwired: 1 in, 2 out]
      }
      event "btnSlot_Ch_Power": Value Change {
        n247 = event-data() -> ()  [unwired: 1 in, 1 out]
        n248 = Enqueue Element(queue=w449, element="btnSlot_Ch_Power" ("元素"), error in (no error)=w448) -> (error out=w450:errorcluster)  [unwired: 1 in, 2 out]
      }
      event "btnSlot_Power": Value Change {
        n249 = event-data() -> ()  [unwired: 1 in, 1 out]
        n250 = Enqueue Element(queue=w453, element="btnSlot_Power" ("元素"), error in (no error)=w452) -> (error out=w454:errorcluster)  [unwired: 1 in, 2 out]
      }
      event "btnZeroing": Value Change {
        n251 = event-data() -> ()  [unwired: 1 in, 1 out]
        n252 = Enqueue Element(queue=w457, element="btnZeroing" ("元素"), error in (no error)=w456) -> (error out=w458:errorcluster)  [unwired: 1 in, 2 out]
      }
      event "btnGetWavelength": Value Change {
        n253 = event-data() -> ()  [unwired: 1 in, 1 out]
        n254 = Enqueue Element(queue=w461, element="btnGetWavelength" ("元素"), error in (no error)=w460) -> (error out=w462:errorcluster)  [unwired: 1 in, 2 out]
      }
      event "btnGetError": Value Change {
        n255 = event-data() -> ()  [unwired: 1 in, 1 out]
        n256 = Enqueue Element(queue=w465, element="btnGetError" ("元素"), error in (no error)=w464) -> (error out=w466:errorcluster)  [unwired: 1 in, 2 out]
      }
      event "btnGetIP": Value Change {
        n257 = event-data() -> ()  [unwired: 1 in, 1 out]
        n258 = Enqueue Element(queue=w469, element="btnGetIP" ("元素"), error in (no error)=w468) -> (error out=w470:errorcluster)  [unwired: 1 in, 2 out]
      }
      event "btnGetPort": Value Change {
        n259 = event-data() -> ()  [unwired: 1 in, 1 out]
        n260 = Enqueue Element(queue=w473, element="btnGetPort" ("元素"), error in (no error)=w472) -> (error out=w474:errorcluster)  [unwired: 1 in, 2 out]
      }
      event "btnSetConst": Value Change {
        n261 = event-data() -> ()  [unwired: 1 in, 1 out]
        n262 = Enqueue Element(queue=w477, element="btnSetConst" ("元素"), error in (no error)=w476) -> (error out=w478:errorcluster)  [unwired: 1 in, 2 out]
      }
      event "btnSetSweep": Value Change {
        n263 = event-data() -> ()  [unwired: 1 in, 1 out]
        n264 = Enqueue Element(queue=w481, element="btnSetSweep" ("元素"), error in (no error)=w480) -> (error out=w482:errorcluster)  [unwired: 1 in, 2 out]
      }
      event "btnSetFreerun": Value Change {
        n265 = event-data() -> ()  [unwired: 1 in, 1 out]
        n266 = Enqueue Element(queue=w485, element="btnSetFreerun" ("元素"), error in (no error)=w484) -> (error out=w486:errorcluster)  [unwired: 1 in, 2 out]
      }
      event "btnStart": Value Change {
        n267 = event-data() -> ()  [unwired: 1 in, 1 out]
        n268 = Enqueue Element(queue=w489, element="btnStart" ("元素"), error in (no error)=w488) -> (error out=w490:errorcluster)  [unwired: 1 in, 2 out]
      }
      event "btnStatus": Value Change {
        n269 = event-data() -> ()  [unwired: 1 in, 1 out]
        n270 = Enqueue Element(queue=w493, element="btnStatus" ("元素"), error in (no error)=w492) -> (error out=w494:errorcluster)  [unwired: 1 in, 2 out]
      }
      event "btnStop": Value Change {
        n271 = event-data() -> ()  [unwired: 1 in, 1 out]
        n272 = Enqueue Element(queue=w497, element="btnStop" ("元素"), error in (no error)=w496) -> (error out=w498:errorcluster)  [unwired: 1 in, 2 out]
      }
      event "btnGetch": Value Change {
        n273 = event-data() -> ()  [unwired: 1 in, 1 out]
        n274 = Enqueue Element(queue=w501, element="btnGetch" ("元素"), error in (no error)=w500) -> (error out=w502:errorcluster)  [unwired: 1 in, 2 out]
      }
      event "btnGetSlot": Value Change {
        n275 = event-data() -> ()  [unwired: 1 in, 1 out]
        n276 = Enqueue Element(queue=w505, element="btnGetSlot" ("元素"), error in (no error)=w504) -> (error out=w506:errorcluster)  [unwired: 1 in, 2 out]
      }
      event "btnGetParameter": Value Change {
        n277 = event-data() -> ()  [unwired: 1 in, 1 out]
        n278 = Enqueue Element(queue=w509, element="btnGetParameter" ("元素"), error in (no error)=w508) -> (error out=w510:errorcluster)  [unwired: 1 in, 2 out]
      }
      event "btnVisa": Value Change {
        n279 = event-data() -> ()  [unwired: 1 in, 1 out]
        n280 = Enqueue Element(queue=w513, element="btnVisa" ("元素"), error in (no error)=w512) -> (error out=w514:errorcluster)  [unwired: 1 in, 2 out]
      }
      event "Communication": Value Change {
        n281 = event-data() -> ()  [unwired: 1 in, 1 out]
        n282 = Enqueue Element(queue=w517, element="Communication" ("元素"), error in (no error)=w516) -> (error out=w518:errorcluster)  [unwired: 1 in, 2 out]
      }
      event Panel Close {
        n283 = event-data() -> ()  [unwired: 1 in, 1 out]
      }
    }
    n284 = Unbundle By Name(w395) -> ("status"=w398:bool)
    n285 = Or(x=w398, y=w397) -> (x .or. y?=w396:bool)
  }
  n286 = Release Queue(queue=w1, error in (no error)=w5) -> ()  [unwired: 1 in, 3 out]
